vi "time2mm.vi"(1 "fs[1]/ps[0]":bool=TRUE, 2 "Offset (mm)":dbl, 3 "time":dbl) -> (0 "position (mm)":dbl)   [LabVIEW 2020]
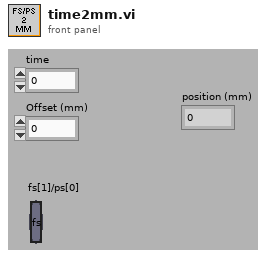
[diagram p1: front panel]
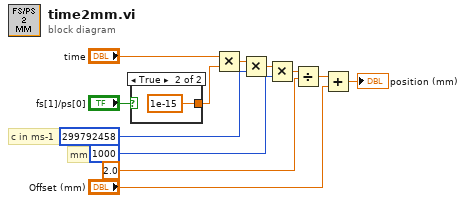
[diagram p0: block diagram]
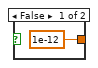
[diagram p2: hidden frame]
diagram:
  # "mm"
  # "c in ms-1"
  n1 = case shown="True" "fs[1]/ps[0]" {
    tunnel: [1e-12 ("y") 1e-15 ("y")] -> w8
    frame False {
    }
    frame True {
    }
  }
  n2 = Multiply(x="time", y=w8) -> (x*y=w2:dbl)
  n3 = Multiply(x=w2, y=299792458) -> (x*y=w4:dbl)
  n4 = Multiply(x=w4, y=1000) -> (x*y=w6:dbl)
  n5 = Divide(x=w6, y=2.0) -> (x/y=w9:dbl)
  n6 = Add(x=w9, y="Offset (mm)") -> (x+y=→"position (mm)":dbl)
